vi "make_histogram.vi"(1 "# intervals (mutli-shot)":i32=128, 2 "Array of ROI sums":dbl[][][][](array[numeric]), 3 "Photoelectron Scaling":dbl=5.8) -> (0 "Histogram over all images, for each region":T1(array[cluster]))   [LabVIEW 2013]
uses:
  <vilib>/Analysis/NI_AALBase.lvlib
panel:
  out "Histogram of ROI Sum over All Images":T2(graph)
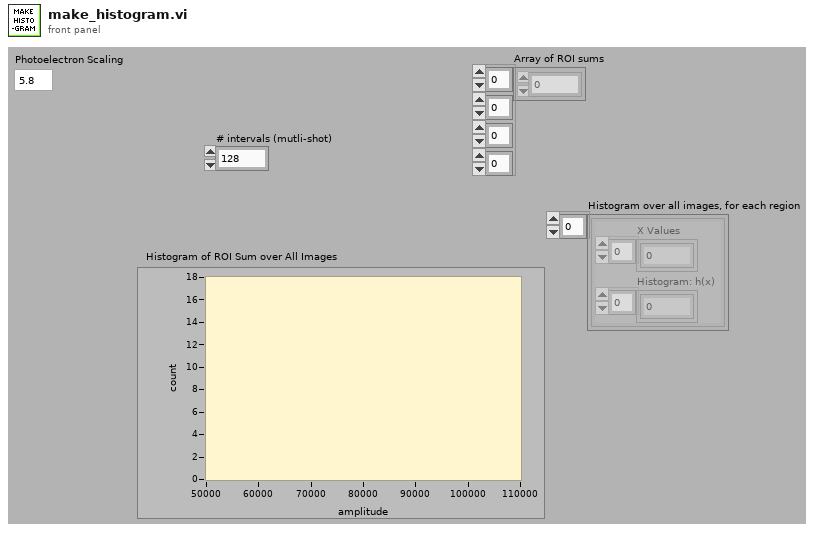
[diagram p1: front panel]
types:
  T1 = cluster{"X Values":dbl[], "Histogram: h(x)":i32[]}[]
  T2 = cluster{"X Values":dbl[], "Histogram: h(x)":i32[]}
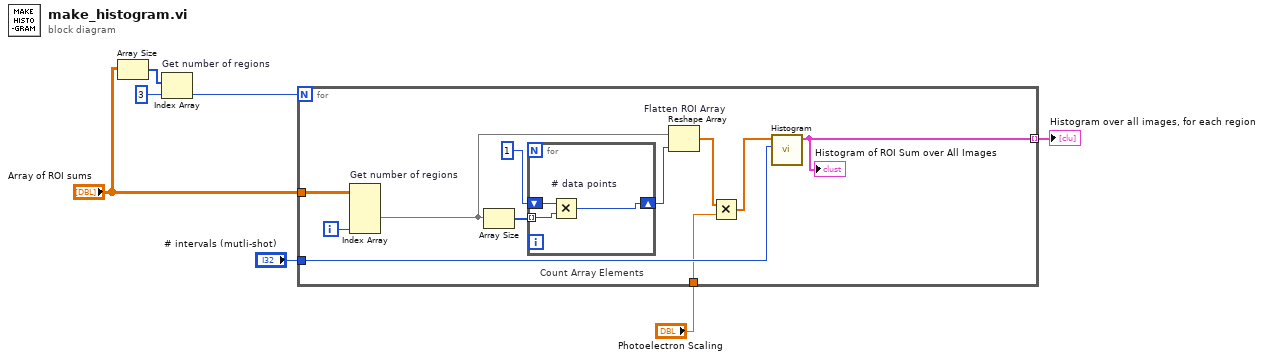
[diagram p0: block diagram]
diagram:
  n1 = Array Size(array="Array of ROI sums") -> (size(s)=w5:i32[])
  n2 = Index Array "Get number of regions"(array=w5, index=3) -> (element=w3:i32)
  n3 = for {
    N: w3 -> [_]
    tunnel: "# intervals (mutli-shot)" -> [w18]
    tunnel: "Array of ROI sums" -> [w14]
    tunnel: [w11] -> w2 mode=indexing
    tunnel: "Photoelectron Scaling" -> [w10]
    i -> [w12]
    n4 = Index Array "Get number of regions"(array=w14, index (dim 3)=w12) -> (element=w13:dbl[][][])  [unwired: 3 in]
    n5 = Array Size(array=w13) -> (size(s)=w17:i32[])
    n6 = for "Count Array Elements" {
      tunnel: w17 -> [w21] mode=indexing
      shift-right: [w19] -> w15
      shift-left: 1 -> [w20]
      n7 = Multiply "# data points"(x=w20, y=w21) -> (x*y=w19:i32)
    }
    n8 = Reshape Array "Flatten ROI Array"(w13, w15) -> (w9:dbl[])
    n9 = Multiply(x=w9, y=w10) -> (x*y=w8:dbl[])
    n10 = call <vilib>:"Histogram.vi"("intervals"=w18, "X"=w8) -> ("Histogram Graph"=w11:T2)  [unwired: 6 in, 3 out]
    "Histogram of ROI Sum over All Images" <- w11
  }
  "Histogram over all images, for each region" <- w2
